vi "DynamicLoadNewGraph.vi"(7 "ViewerPath":path, 8 "error in (no error)":errorcluster, 10 "Preferred_tags":string[](array[string]), 11 "Gserver in":refnum<class "Gserver.lvclass">) -> (0 "error out":errorcluster, 3 "Gserver out":refnum<class "Gserver.lvclass">)   [LabVIEW 2020, in "Sgraph_lib_V1.lvlib" / "Gserver.lvclass"]
doc: "Andre Koelewijn, 2 jan 2021\n\nDynamically open a new Gviewer application instance.\nThe name of the new instance depends upon the numbers of open graphs and is determined by Gserver.\nThe maximum number of allowed graphs is defined as provided to this vi."
uses:
  Gserver.lvclass
  Gserver.lvclass/Gserver.ctl
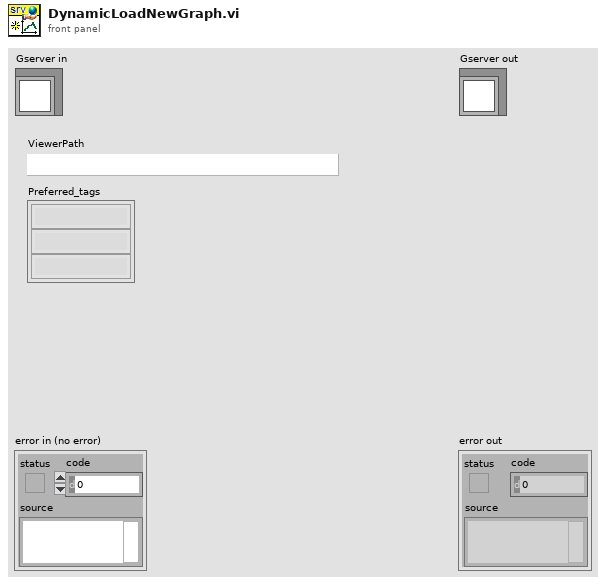
[diagram p1: front panel]
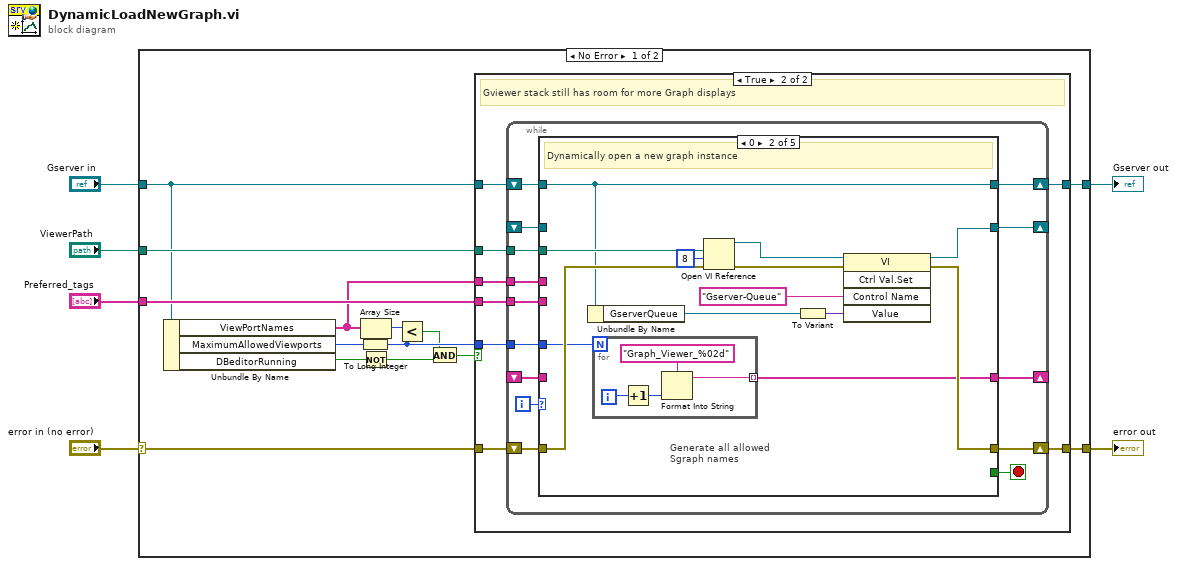
[diagram p0: block diagram]
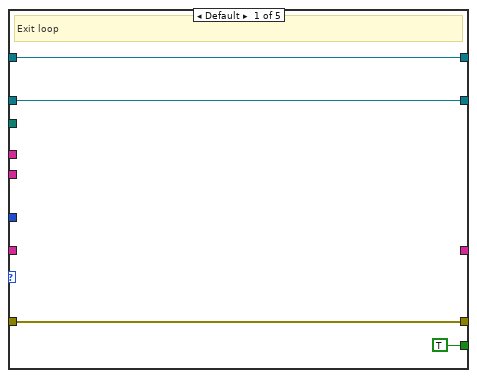
[diagram p3: hidden frame]
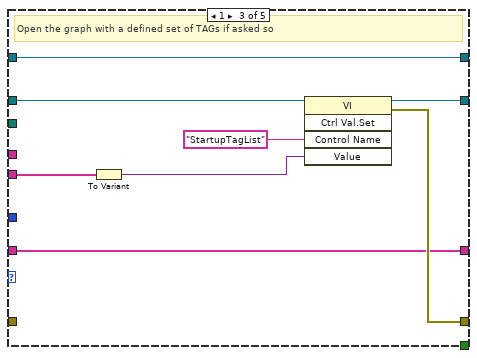
[diagram p4: hidden frame]
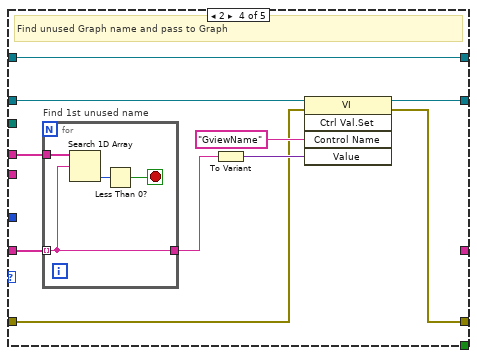
[diagram p5: hidden frame]
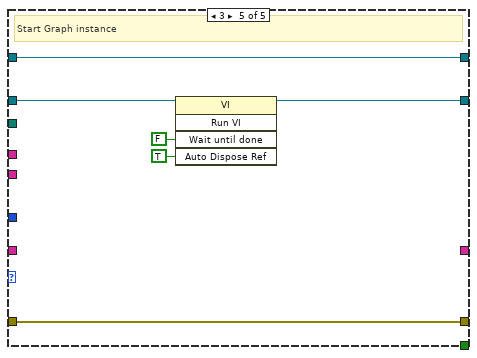
[diagram p6: hidden frame]
diagram:
  n1 = case shown="No Error" "error in (no error)" {
    selector: "error in (no error)" -> [w19 w95]
    tunnel: [w15 w95] -> w5
    tunnel: [w18 w94] -> w3
    tunnel: "Gserver in" -> [w16 w94]
    tunnel: "ViewerPath" -> [w20 _]
    tunnel: "Preferred_tags" -> [w17 _]
    frame No Error {
      n2 = Unbundle By Name(w16) -> ("ViewPortNames"=w11:string[], "MaximumAllowedViewports"=w13:u8, "DBeditorRunning"=w9:bool)
      n3 = To Long Integer(number=w13) -> (32bit integer=w12:i32)
      n4 = Array Size(array=w11) -> (size(s)=w14:i32)
      n5 = Not(x=w9) -> (.not. x?=w8:bool)
      n6 = Less?(x=w14, y=w12) -> (x < y?=w10:bool)
      n7 = And(x=w10, y=w8) -> (x .and. y?=w7:bool)
      n8 = case shown="True" w7 {
        tunnel: w20 -> [_ w30]
        tunnel: w19 -> [w21 w29]
        tunnel: [w22 w28] -> w18
        tunnel: w17 -> [_ w27]
        tunnel: w16 -> [w22 w26]
        tunnel: [w21 w25] -> w15
        tunnel: w12 -> [_ w24]
        tunnel: w11 -> [_ w23]
        frame False {
          # "Maximum number of Graph displays is reached"
        }
        frame True {
          # "Gviewer stack still has room for more Graph displays"
          n9 = while {
            tunnel: w30 -> [w44]
            shift-right: [w40] -> w28
            shift-left: w26 -> [w41]
            shift-right: [w38] -> w25
            shift-left: w29 -> [w43]
            shift-right: [w39] -> _
            shift-left: _ -> [w37]
            tunnel: w27 -> [w35]
            tunnel: w24 -> [w34]
            shift-right: [w33] -> _
            shift-left: _ -> [w32]
            tunnel: w23 -> [w31]
            i -> [w42]
            stop <- w36 stop-if-true
            n10 = case shown="0" w42 {
              tunnel: w44 -> [_ w61 _ _ _]
              tunnel: w43 -> [w46 w60 _ w77 w92]
              tunnel: w41 -> [w47 w57 w72 w82 w93]
              tunnel: [w47 w57 w72 w82 w93] -> w40
              tunnel: [w48 w52 w69 w79 w88] -> w39
              tunnel: [w46 w53 w70 w80 w92] -> w38
              tunnel: w37 -> [w48 _ w68 w78 w91]
              tunnel: [TRUE _ _ _ _] -> w36
              tunnel: w35 -> [_ _ w67 _ _]
              tunnel: w34 -> [_ w50 _ _ _]
              tunnel: [_ w49 w66 _ _] -> w33
              tunnel: w32 -> [_ _ w66 w75 _]
              tunnel: w31 -> [_ _ _ w76 _]
              frame Default {
                # "Exit loop"
              }
              frame 0 {
                # "Generate all allowed\nSgraph names"
                # "Dynamically open a new graph instance"
                n11 = Unbundle By Name(w57) -> ("GserverQueue"=w56:refnum<queue>)
                n12 = for {
                  N: w50 -> [_]
                  tunnel: [w62] -> w49 mode=indexing
                  i -> [w64]
                  n13 = Increment(x=w64) -> (x+1=w63:i32)
                  n14 = Format Into String(format string="Graph_Viewer_%02d" ("Control Name"), w63) -> (resulting string=w62:string)  [unwired: 2 in, 1 out]
                }
                n15 = Open VI Reference(vi path=w61, options=8, error in (no error)=w60) -> (vi reference=w58:refnum<vi>, error out=w54:errorcluster)  [unwired: 3 in]
                n16 = To Variant(anything=w56) -> (Variant=w55:variant)
                n17 = invoke class="VI" method="Ctrl Val.Set"(reference=w58, error in=w54, "Control Name"="Gserver-Queue", "Value"=w55) -> (reference out=w52:refnum<vi>, error out=w53:errorcluster)  [unwired: 1 in, 3 out]
              }
              frame 1 {
                # "Open the graph with a defined set of TAGs if asked so"
                n18 = To Variant(anything=w67) -> (Variant=w71:variant)
                n19 = invoke class="VI" method="Ctrl Val.Set"(reference=w68, "Control Name"="StartupTagList", "Value"=w71) -> (reference out=w69:refnum<vi>, error out=w70:errorcluster)  [unwired: 2 in, 3 out]
              }
              frame 2 {
                # "Find unused Graph name and pass to Graph"
                n20 = for "Find 1st unused name" {
                  tunnel: w75 -> [w84] mode=indexing
                  tunnel: w76 -> [w85]
                  tunnel: [w84] -> w74
                  stop <- w86 stop-if-true
                  n21 = Search 1D Array(1D array=w85, element=w84) -> (index of element=w87:i32)  [unwired: 1 in]
                  n22 = Less Than 0?(x=w87) -> (x < 0?=w86:bool)
                }
                n23 = To Variant(anything=w74) -> (Variant=w81:variant)
                n24 = invoke class="VI" method="Ctrl Val.Set"(reference=w78, error in=w77, "Control Name"="GviewName", "Value"=w81) -> (reference out=w79:refnum<vi>, error out=w80:errorcluster)  [unwired: 1 in, 3 out]
              }
              frame 3 {
                # "Start Graph instance"
                n25 = invoke class="VI" method="Run VI"(reference=w91, "Wait until done"=FALSE ("Wait Until Done"), "Auto Dispose Ref"=TRUE ("Auto Dispose Reference")) -> (reference out=w88:refnum<vi>)  [unwired: 2 in, 4 out]
              }
            }
          }
        }
      }
    }
    frame Error {
    }
  }
  "error out" <- w5
  "Gserver out" <- w3
